vi "Create Message Log ID.vi"(10 "IP Address":string, 11 "Head Worker WID":string) -> (3 "Message Log ID":T1)   [LabVIEW 2017]
uses:
  Message Log ID.ctl
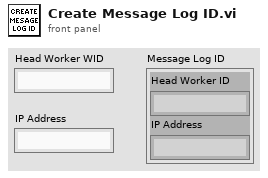
[diagram p1: front panel]
types:
  T1 = typedef "Message Log ID.ctl" = cluster{"Head Worker ID":string, "IP Address":string}
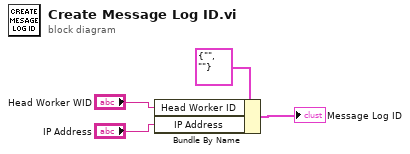
[diagram p0: block diagram]
diagram:
  n1 = Bundle By Name(cluster=T1 {"Head Worker ID"="", "IP Address"=""} ("ML_ID"), "Head Worker ID"="Head Worker WID", "IP Address"="IP Address") -> (→"Message Log ID":T1)
